vi "Test App Removed Process Lifecycle Not Managed by App.vi"(8 "error in (no error)":errorcluster, 11 "Rig Test in":refnum<class "Application Dev Test.lvclass">) -> (0 "error out":errorcluster, 3 "Rig Test out":refnum<class "Application Dev Test.lvclass">)   [LabVIEW 2020, in "Application Dev Test.lvclass"]
uses:
  Application Dev Test.lvclass
  C:/Program Files (x86)/National Instruments/LabVIEW 2020/vi.lib/Astemes/LUnit/Test Case.lvclass
  source/Framework/Process/Process.lvclass
  source/Framework/Process/Public/Lifecycle/Lifecycle State.ctl
  source/Framework/Process/Process.lvclass/Process.ctl
  source/Framework/Application/Application.lvclass/Application.ctl
  <vilib>/Astemes/LUnit/Test Case.lvclass/Test Case.ctl
  source/Framework/Application/Private/Add Process to Map.vi
  source/Framework/Application/Private/Throw Error If Process Already in App.vi
  source/Framework/Process/Protected/Messaging/Send Message.vi
  source/Framework/Process/Protected/SubVIs/Set Context.vi
  source/Framework/Application/Private/Remove Process from App.vi
  source/Framework/Application/Private/Parse Process Name.vi
  source/Framework/Application/Private/Remove Process from Map.vi
  source/Framework/Process/Protected/SubVIs/Clear Context.vi
  source/Framework/Process/Private/SubVIs/Wait for finish.vi
  source/Framework/Process/Private/SubVIs/Set Lifecycle State.vi
  <vilib>/Utility/error.llb/Clear Errors.vi
  <vilib>/Astemes/LUnit/Palette/Fail.vi
  <vilib>/Astemes/LUnit/Palette/Pass.vi
  <vilib>/Astemes/LUnit/Set Assertion Type.vi
  source/Framework/Application/Public/Get Process.vi
  source/Framework/Process/Private/SubVIs/Handle Debug Data.vi
  source/Framework/Process/Public/Lifecycle/Leave Process Loop.vi
  source/Framework/Process/Protected/Messaging/Request Message.vi
  <vilib>/AdvancedString/Delimited String to 1D String Array.vi
  <vilib>/Astemes/LUnit/Add test result.vi
  source/Framework/Application/Private/Retrieve Process from App.vi
  source/Framework/Application/Private/Get Process from Map.vi
  source/Framework/Logging/Log Debug.vi
  <vilib>/AdvancedString/1D String Array to Delimited String.vi
  <vilib>/Utility/High Resolution Relative Seconds.vi
  source/Framework/Process/Private/SubVIs/Enqueue Request Message.vi
  <vilib>/Astemes/LUnit/LUnit Record Assertion Result.vi
  <vilib>/Astemes/LUnit/LUnit Aggregate Assertion Results.vi
  <vilib>/Astemes/LUnit/Method Result/LUnit Merge Status.vi
  <vilib>/Astemes/LUnit/LUnit Concatenate result strings.vi
  source/Framework/Application/Application.lvclass
  C:/Git/astemes-triarc-framework/source/Framework/Process/Process.lvclass
  <vilib>/Utility/error.llb/Error Cluster From Error Code.vi
  source/Framework/Process/Public/Read Name.vi
  source/Framework/Process/Private/SubVIs/Wait for Response Message.vi
  Application Dev Test.lvclass/Application Dev Test.ctl
  C:/Git/astemes-triarc-framework/source/Framework/Base/Base.lvclass
  C:/Git/astemes-triarc-framework/source/Framework/Error Handler Interface/Error Handler Interface.lvclass
  C:/Git/astemes-triarc-framework/source/Framework/Logging/Logging.lvclass
  C:/Git/astemes-triarc-framework/source/Framework/Application/Application.lvclass
  C:/Git/astemes-triarc-framework/source/Framework/Async Handler/Async Handler.lvclass
  <vilib>/Astemes/LUnit/Test Case.lvclass
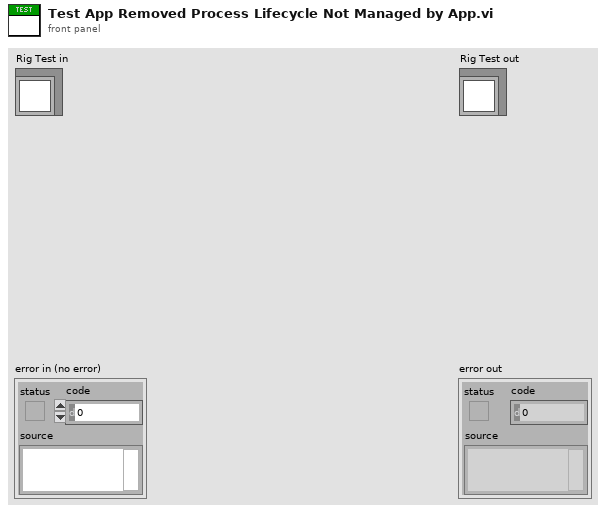
[diagram p1: front panel]
types:
  T1 = typedef "Process.lvclass/Lifecycle State.ctl" = enum16{"Uninitialized", "Initialized", "Started", "Running", "Stopped", "Finished"}
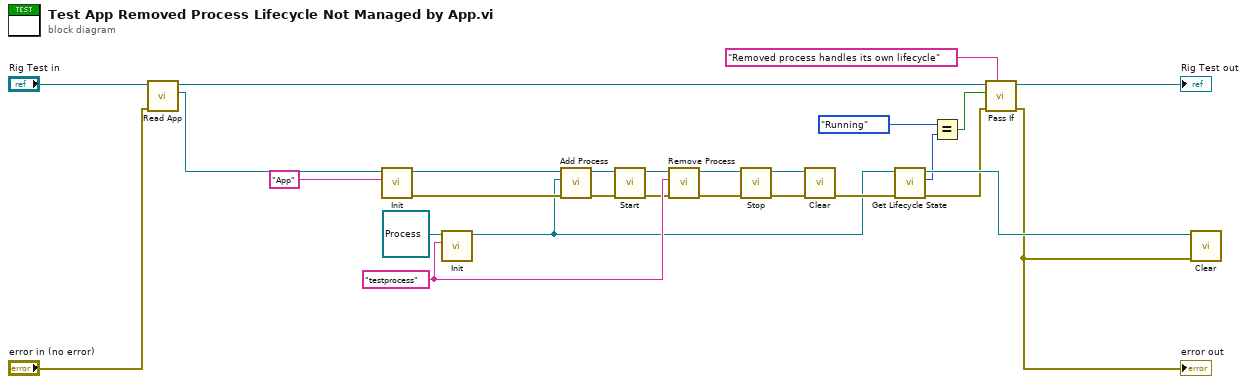
[diagram p0: block diagram]
diagram:
  w11 = "testprocess" ("Name")
  n1 = call "Read App.vi"("error in (no error)"="error in (no error)", "Application Test In"="Rig Test in") -> ("App out"=w26:refnum<class "Application.lvclass">, "Application Test Out"=w18:refnum<class "Application Dev Test.lvclass">)  [unwired: 7 in, 1 out]
  n2 = call-dynamic "Init.vi"("Name"="App", "Process In"=w26) -> ("error out"=w19:errorcluster, "Process Out"=w20:refnum<class "Application.lvclass">)  [unwired: 8 in]
  n3 = call-dynamic "Init.vi"("Name"=w11, "Process In"=refnum<class "Process.lvclass"> refnum ("Process.lvclass")) -> ("Process Out"=w4:refnum<class "Process.lvclass">)  [unwired: 8 in, 1 out]
  n4 = call "Add Process.vi"("error in (no error)"=w19, "Process"=w4, "Application In"=w20) -> ("error out"=w23:errorcluster, "Application Out"=w2:refnum<class "Application.lvclass">)  [unwired: 7 in]
  n5 = call "Start.vi"("error in (no error)"=w23, "Process In"=w2) -> ("error out"=w3:errorcluster, "Process Out"=w1:refnum<class "Application.lvclass">)  [unwired: 7 in, 1 out]
  n6 = call "Remove Process.vi"("error in (no error)"=w3, "Process Name"=w11, "Application In"=w1) -> ("error out"=w14:errorcluster, "Application Out"=w13:refnum<class "Application.lvclass">)  [unwired: 6 in, 1 out]
  n7 = call "Stop.vi"("error in (no error)"=w14, "Process In"=w13) -> ("error out"=w16:errorcluster, "Process Out"=w15:refnum<class "Application.lvclass">)  [unwired: 7 in, 1 out]
  n8 = call-dynamic "Clear.vi"("error in (no error)"=w16, "Application In"=w15) -> ("error out"=w12:errorcluster)  [unwired: 9 in]
  n9 = call "Get Lifecycle State.vi"("error in (no error)"=w12, "Process In"=w4) -> ("error out"=w9:errorcluster, "Lifecycle State"=w7:T1, "Process Out"=w10:refnum<class "Process.lvclass">)  [unwired: 6 in, 1 out]
  n10 = Equal?(x=Lifecycle_State."Running" ("Lifecycle State"), y=w7) -> (x = y?=w5:bool)
  n11 = call <vilib>:"Pass If.vi"("Description"="Removed process handles its own lifecycle", "error in (no error)"=w9, "Pass?"=w5, "LUnit Test Case In"=w18) -> ("error out"=w8:errorcluster, "LUnit Test Case Out"=→"Rig Test out":refnum<class "Application Dev Test.lvclass">)  [unwired: 6 in]
  "error out" <- w8
  n12 = call-dynamic "Clear.vi"("error in (no error)"=w8, "Process In"=w10) -> ()  [unwired: 9 in, 1 out]
